vi "Apply Material Information.vi"(6 "Materials":T1(array[cluster]), 7 "Load Material Textures":bool, 8 "error in (no error)":errorcluster, 9 "material_id":i32, 10 "Material Path":path, 11 "SceneObject in":refnum<vi>) -> (0 "error out":errorcluster, 3 "SceneObject out":refnum<vi>)   [LabVIEW 2020, in "g_ar_toolkit.ar.lvlib"]
uses:
  g_ar_toolkit.ar.lvlib
  <vilib>/Utility/miscctls.llb/LVRGBAColorTypeDef.ctl
  <vilib>/picture/3D Picture Control/Helpers/Apply Texture (no reference).vi
  <vilib>/picture/3D Picture Control/NI_3D Picture Control.lvlib
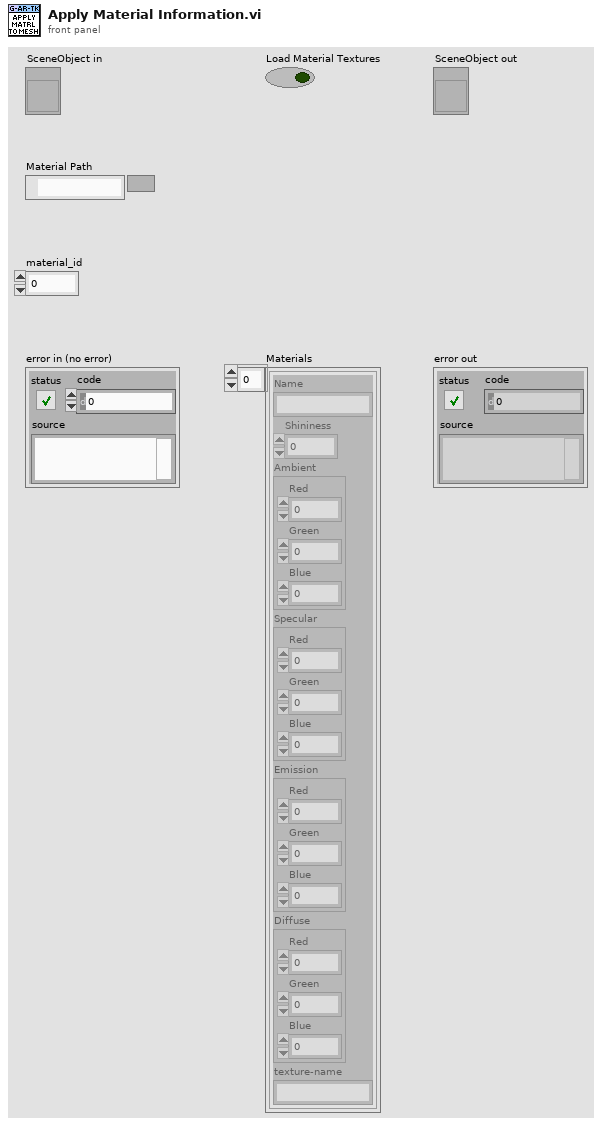
[diagram p1: front panel]
types:
  T1 = cluster{"Name":string, "Shininess":sgl, "Ambient":cluster{"Red":sgl, "Green":sgl, "Blue":sgl}, "Specular":cluster{"Red":sgl, "Green":sgl, "Blue":sgl}, "Emission":cluster{"Red":sgl, "Green":sgl, "Blue":sgl}, "Diffuse":cluster{"Red":sgl, "Green":sgl, "Blue":sgl}, "texture-name":string}[]
  T2 = enum16{"Inherit Material", "Use entire Material", "Ignore Ambient", "Ignore Diffuse", "Ignore Specular", "Ignore Emission", "Ignore Ambient and Diffuse"}
  T3 = typedef "LVRGBAColorTypeDef.ctl" = cluster{"Red":sgl, "Green":sgl, "Blue":sgl, "Alpha":sgl}
  T4 = cluster{"Name":string, "Shininess":sgl, "Ambient":cluster{"Red":sgl, "Green":sgl, "Blue":sgl}, "Specular":cluster{"Red":sgl, "Green":sgl, "Blue":sgl}, "Emission":cluster{"Red":sgl, "Green":sgl, "Blue":sgl}, "Diffuse":cluster{"Red":sgl, "Green":sgl, "Blue":sgl}, "texture-name":string}
  T5 = typedef "imagedata.ctl" = cluster{"image type":i32, "image depth":i32, "image":u8[], "mask":u8[], "colors":u32[], "Rectangle":cluster{"left":i16, "top":i16, "right":i16, "bottom":i16}}
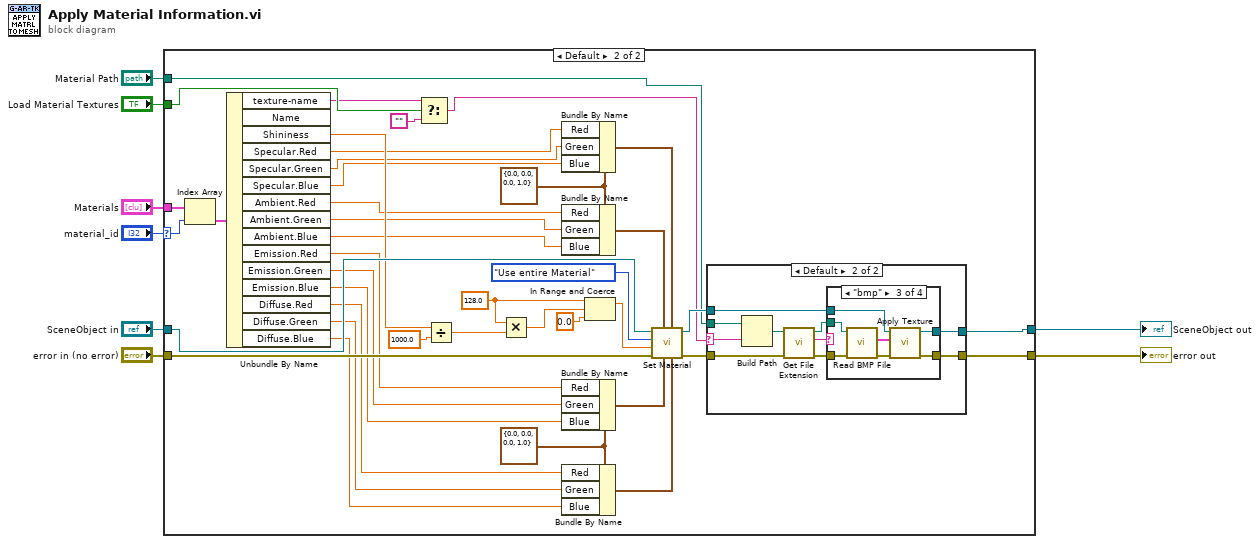
[diagram p0: block diagram]
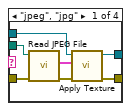
[diagram p4: hidden frame]
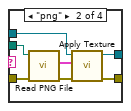
[diagram p5: hidden frame]
diagram:
  n1 = case shown="Default" "material_id" {
    selector: "material_id" -> [_ w40]
    tunnel: "SceneObject in" -> [w9 w50]
    tunnel: [w9 w38] -> w1
    tunnel: "error in (no error)" -> [w10 w49]
    tunnel: [w10 w36] -> w2
    tunnel: "Materials" -> [_ w47]
    tunnel: "Material Path" -> [_ w34]
    tunnel: "Load Material Textures" -> [_ w30]
    frame -1 {
    }
    frame Default {
      w13 = T3 {"Red"=0.0, "Green"=0.0, "Blue"=0.0, "Alpha"=1.0} ("Color")
      w17 = T3 {"Red"=0.0, "Green"=0.0, "Blue"=0.0, "Alpha"=1.0} ("Color")
      w42 = sgl 128.0 ("upper limit")
      n2 = Index Array(array=w47, index=w40) -> (element=w35:T4)
      n3 = Unbundle By Name(w35) -> ("texture-name"=w11:string, "Shininess"=w46:sgl, "Specular.Red"=w29:sgl, "Specular.Green"=w28:sgl, "Specular.Blue"=w27:sgl, "Ambient.Red"=w25:sgl, "Ambient.Green"=w24:sgl, "Ambient.Blue"=w23:sgl, "Emission.Red"=w21:sgl, "Emission.Green"=w20:sgl, "Emission.Blue"=w19:sgl, "Diffuse.Red"=w16:sgl, "Diffuse.Green"=w15:sgl, "Diffuse.Blue"=w14:sgl)  [unwired: 1 out]
      n4 = Select(t=w11, s=w30, f="") -> (s? t:f=w32:string)
      n5 = Divide(x=w46, y=sgl 1000.0 ("x")) -> (x/y=w45:sgl)
      n6 = Multiply(x=w42, y=w45) -> (x*y=w41:sgl)
      n7 = Bundle By Name(cluster=w17, "Red"=w29, "Green"=w28, "Blue"=w27) -> (w26:T3)
      n8 = Bundle By Name(cluster=w17, "Red"=w25, "Green"=w24, "Blue"=w23) -> (w22:T3)
      n9 = Bundle By Name(cluster=w13, "Red"=w21, "Green"=w20, "Blue"=w19) -> (w18:T3)
      n10 = Bundle By Name(cluster=w13, "Red"=w16, "Green"=w15, "Blue"=w14) -> (w12:T3)
      n11 = In Range and Coerce(upper limit=w42, x=w41, lower limit=sgl 0.0) -> (coerced(x)=w33:sgl)  [unwired: 1 out]
      n12 = call <vilib>:"Set Material.vi"("Diffuse"=w12, "Specular"=w26, "Emission"=w18, "Ambient"=w22, "error in (no error)"=w49, "Shininess"=w33, "Color Mode"=T2."Use entire Material", "Scene Object In"=w50) -> ("error out"=w37:errorcluster, "Scene Object Out"=w39:refnum<vi>)  [unwired: 2 in]
      n13 = case shown="Default" w32 {
        selector: w32 -> [_ w53]
        tunnel: w39 -> [w51 w59]
        tunnel: [w51 w58] -> w38
        tunnel: w37 -> [w52 w56]
        tunnel: [w52 w55] -> w36
        tunnel: w34 -> [_ w54]
        frame "" {
        }
        frame Default {
          n14 = Build Path(base path=w54, name or relative path=w53) -> (appended path=w62:path)
          n15 = call <vilib>:"Get File Extension.vi"("error in (no error)"=w56, "file"=w62) -> ("error out"=w57:errorcluster, "lowercase file extension"=w61:string, "dup file"=w60:path)  [unwired: 5 in, 2 out]
          n16 = case shown="\"bmp\"" w61 {
            tunnel: w60 -> [w69 w76 w83 _]
            tunnel: w59 -> [w68 w75 w82 w85]
            tunnel: [w67 w74 w81 w85] -> w58
            tunnel: w57 -> [w65 w72 w79 w84]
            tunnel: [w63 w70 w77 w84] -> w55
            frame "jpeg", "jpg" {
              n17 = call <vilib>:"Read JPEG File.vi"("error in (no error)"=w65, "path to JPEG file"=w69) -> ("error out"=w64:errorcluster, "image data"=w66:T5)  [unwired: 7 in, 1 out]
              n18 = call-poly <vilib>:"Apply Texture.vi"("error in (no error)"=w64, "Image Data"=w66, "Scene Object In"=w68) -> ("error out"=w63:errorcluster, "Scene Object Out"=w67:refnum<vi>)  [unwired: 7 in]
            }
            frame "png" {
              n19 = call <vilib>:"Read PNG File.vi"("error in (no error)"=w72, "path to PNG file"=w76) -> ("error out"=w71:errorcluster, "image data"=w73:T5)  [unwired: 7 in, 1 out]
              n20 = call-poly <vilib>:"Apply Texture.vi"("error in (no error)"=w71, "Image Data"=w73, "Scene Object In"=w75) -> ("error out"=w70:errorcluster, "Scene Object Out"=w74:refnum<vi>)  [unwired: 7 in]
            }
            frame "bmp" {
              n21 = call <vilib>:"Read BMP File.vi"("error in (no error)"=w79, "path to BMP file"=w83) -> ("error out"=w78:errorcluster, "image data"=w80:T5)  [unwired: 7 in, 1 out]
              n22 = call-poly <vilib>:"Apply Texture.vi"("error in (no error)"=w78, "Image Data"=w80, "Scene Object In"=w82) -> ("error out"=w77:errorcluster, "Scene Object Out"=w81:refnum<vi>)  [unwired: 7 in]
            }
            frame Default {
            }
          }
        }
      }
    }
  }
  "error out" <- w2
  "SceneObject out" <- w1
